vi "RREQ_Packet_To_Processed_Bytes.vi"(3 "error in (no error)":errorcluster, 4 "RREQ Param In":T5, 5 "RREQ Packet In":T1) -> (0 "error out":errorcluster, 1 "Processed Bytes":u8[](array[numeric]), 2 "RREQ Packet Out":T1)   [LabVIEW 2017]
uses:
  Controls/Control Packets/RREQ_Param.ctl
  Controls/Packet/Packet.ctl
  Controls/Packet/Packet_Direction.ctl
  Controls/Packet/Packet_Type.ctl
  Controls/Packet/Packet_Priority.ctl
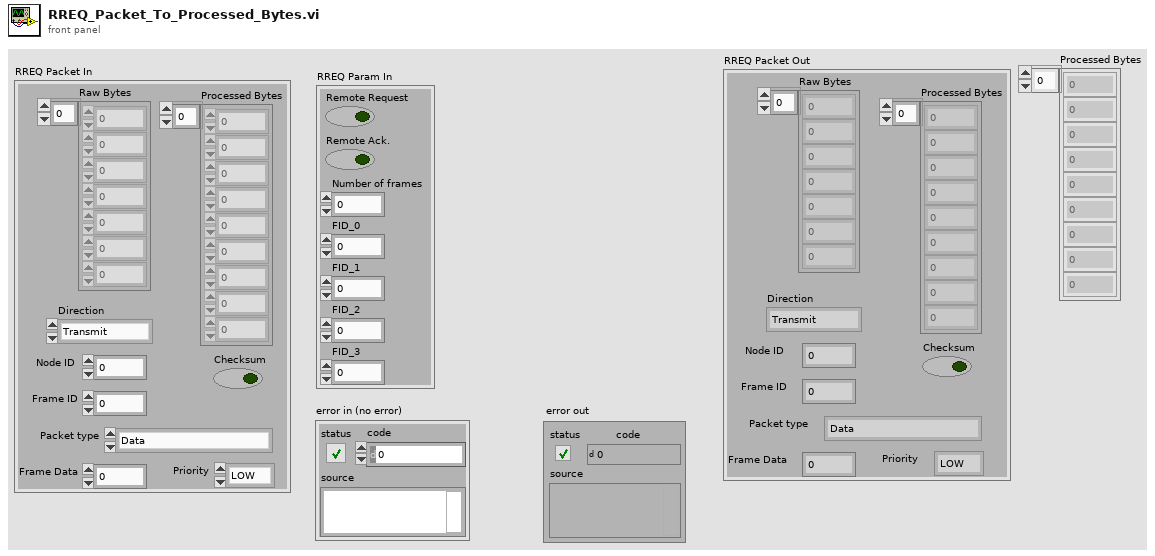
[diagram p1: front panel]
types:
  T1 = typedef "Packet.ctl" = cluster{"Raw Bytes":u8[], "Checksum":bool, "Direction":T2, "Processed Bytes":u8[], "Node ID":u8, "Packet type":T3, "Frame Data":u32, "Priority":T4, "Frame ID":u8}
  T2 = typedef "Packet_Direction.ctl" = enum16{"Transmit", "Receive", "Bidirectional"}
  T3 = typedef "Packet_Type.ctl" = enum16{"Data", "Connection Management", "Remote Request", "Error/Status"}
  T4 = typedef "Packet_Priority.ctl" = enum16{"LOW", "HIGH"}
  T5 = typedef "RREQ_Param.ctl" = cluster{"Remote Request":bool, "Remote Ack.":bool, "Number of frames":u8, "FID_0":u8, "FID_1":u8, "FID_2":u8, "FID_3":u8}
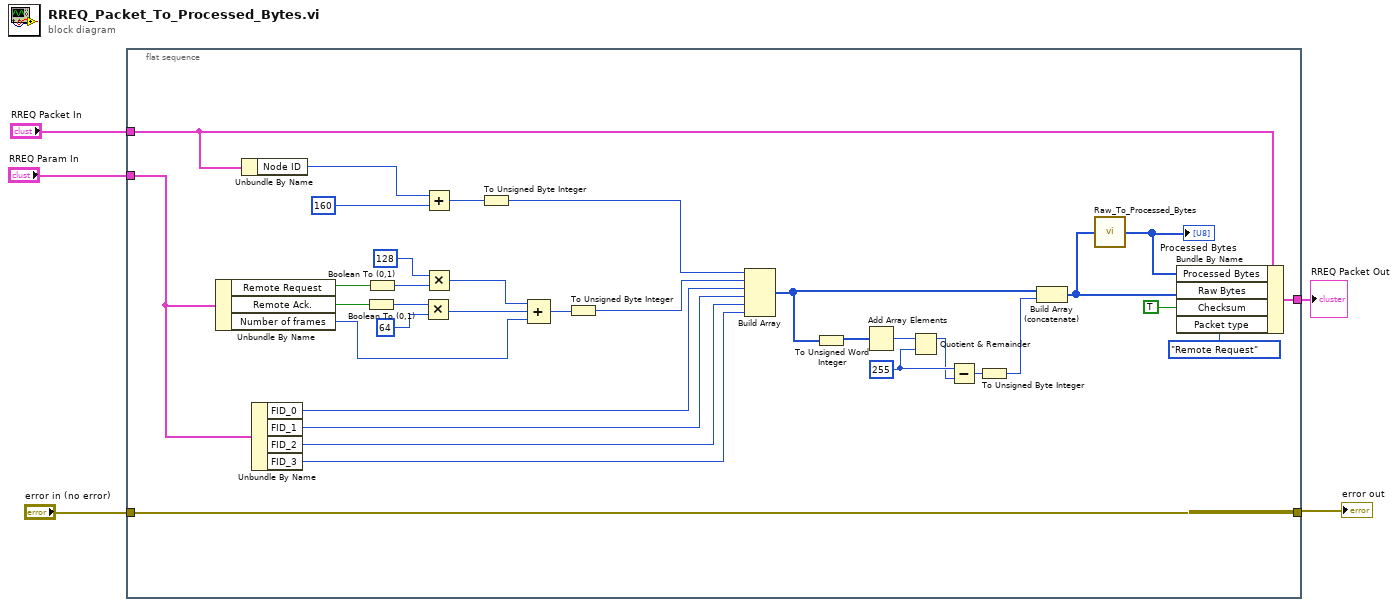
[diagram p0: block diagram]
diagram:
  n1 = flat-sequence {
    tunnel: "error in (no error)" -> [w39]
    tunnel: [w39] -> w4
    tunnel: "RREQ Packet In" -> [w11]
    tunnel: "RREQ Param In" -> [w23]
    tunnel: [w7] -> w1
    frame #0 {
      w16 = u16 255 ("y")
      n2 = Unbundle By Name(w23) -> ("Remote Request"=w38:bool, "Remote Ack."=w37:bool, "Number of frames"=w30:u8)
      n3 = Unbundle By Name(w11) -> ("Node ID"=w28:u8)
      n4 = Unbundle By Name(w23) -> ("FID_0"=w22:u8, "FID_1"=w21:u8, "FID_2"=w20:u8, "FID_3"=w19:u8)
      n5 = Boolean To (0,1)(Boolean=w37) -> (0, 1=w34:i16)
      n6 = Boolean To (0,1)(Boolean=w38) -> (0, 1=w36:i16)
      n7 = Multiply(x=w34, y=i16 64) -> (x*y=w31:i16)
      n8 = Add(x=w28, y=u8 160) -> (x+y=w26:u8)
      n9 = Multiply(x=i16 128, y=w36) -> (x*y=w32:i16)
      n10 = To Unsigned Byte Integer(number=w26) -> (unsigned 8bit integer=w25:u8)
      n11 = Compound Arithmetic op=ADD(w32, w31, w30) -> (w29:i16)
      n12 = To Unsigned Byte Integer(number=w29) -> (unsigned 8bit integer=w24:u8)
      n13 = Build Array(w25, w24, w22, w21, w20, w19) -> (w12:u8[])
      n14 = To Unsigned Word Integer(number=w12) -> (unsigned 16bit integer=w18:u16[])
      n15 = Add Array Elements(numeric array=w18) -> (sum=w17:u16)
      n16 = Quotient & Remainder(x=w17, y=w16) -> (x-y*floor(x/y)=w15:u16)  [unwired: 1 out]
      n17 = Subtract(x=w16, y=w15) -> (x-y=w14:u16)
      n18 = To Unsigned Byte Integer(number=w14) -> (unsigned 8bit integer=w13:u8)
      n19 = Build Array (concatenate)(w12, w13) -> (w6:u8[])
      n20 = call "Raw_To_Processed_Bytes.vi"("Raw Bytes"=w6) -> ("Processed Bytes"=w10:u8[])
      "Processed Bytes" <- w10
      n21 = Bundle By Name(cluster=w11, "Processed Bytes"=w10, "Raw Bytes"=w6, "Checksum"=TRUE, "Packet type"=Packet_Type."Remote Request") -> (w7:T1)
    }
  }
  "error out" <- w4
  "RREQ Packet Out" <- w1
